vi "Test 1.vi"() -> ()   [LabVIEW 2012, in "Universal Power Meter.lvlib"]
uses:
  Universal Power Meter.lvlib
  <vilib>/ActorFramework/Message Queue/Message Queue.lvclass/Message Queue.ctl
  <vilib>/ActorFramework/Message Enqueuer/Message Enqueuer.lvclass/Message Enqueuer.ctl
  <vilib>/ActorFramework/Message Enqueuer/Enqueue.vi
  <vilib>/ActorFramework/Message Priority Queue/Priority Enqueue.vi
  <vilib>/ActorFramework/Stop Msg/Stop Msg.lvclass
  <vilib>/ActorFramework/Message Queue/Message Queue.lvclass
  <vilib>/ActorFramework/Actor/Actor.lvclass
  Universal Power Meter.lvclass
panel:
  in  "VISA resource name":refnum<visa-resource-name>="GPIB0::21::INSTR"
  out "Numeric Control":i32
  in  "Stop Button":bool
  out "error out":errorcluster
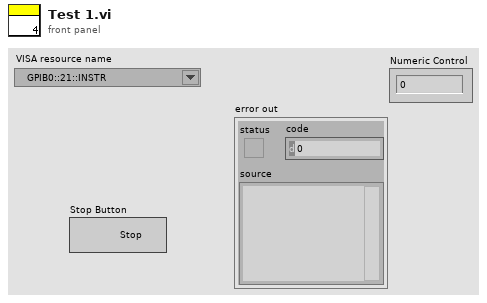
[diagram p1: front panel]
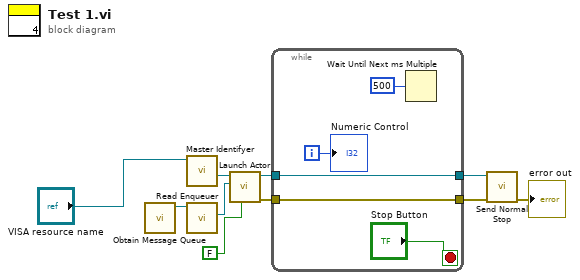
[diagram p0: block diagram]
diagram:
  n1 = call <vilib>:"Obtain Message Queue.vi"() -> ("Message Queue"=w10:refnum<class "Message Queue.lvclass">)  [unwired: 10 in, 1 out]
  n2 = call "Master Identifyer.vi"("VISA resource name"="VISA resource name") -> ("Class out"=w1:refnum<class "Universal Power Meter.lvclass">)  [unwired: 10 in]
  n3 = call <vilib>:"Read Enqueuer.vi"("Message Queue"=w10) -> ("Message Enqueuer"=w9:refnum<class "Message Enqueuer.lvclass">)  [unwired: 10 in]
  n4 = call <vilib>:"Launch Actor.vi"("Open Actor Core front panel? (F)"=FALSE, "Actor-to-Caller Enqueuer"=w9, "Actor"=w1) -> ("error out"=w6:errorcluster, "Caller-To-Actor Enqueuer"=w7:refnum<class "Message Enqueuer.lvclass">)  [unwired: 7 in]
  n5 = while {
    tunnel: [w12] -> w5
    tunnel: w7 -> [w12]
    tunnel: [w15] -> w4
    tunnel: w6 -> [w15]
    i -> [w13]
    stop <- "Stop Button" stop-if-true
    n6 = Wait Until Next ms Multiple(millisecond multiple=u32 500) -> ()  [unwired: 1 out]
    "Numeric Control" <- w13
  }
  n7 = call <vilib>:"Send Normal Stop.vi"("error in (no error)"=w4, "Message Enqueuer"=w5) -> ("error out"=→"error out":errorcluster)  [unwired: 9 in]
